vi "Configure Dialog.vi"(8 "error in (no error)":errorcluster, 11 "Configure Sparse Marker [SM] Msg.lvclass":refnum<class "Configure Sparse Marker [SM] Msg.lvclass">) -> (0 "error out":errorcluster, 2 "Ok?":bool, 3 "Configure Sparse Marker [SM] Msg.lvclass":refnum<class "Configure Sparse Marker [SM] Msg.lvclass">)   [LabVIEW 2015, in "CS++Fgen.lvlib" / "Configure Sparse Marker [SM] Msg.lvclass"]
uses:
  Configure Sparse Marker [SM] Msg.lvclass
  Configure Sparse Marker [SM] Msg.lvclass/Configure Sparse Marker [SM] Msg.ctl
panel:
  in  "Indexes Array":i64[](array[numeric])
  in  "Cancel Button":bool
  in  "OK Button":bool
  in  "Destination Terminal":string
  in  "Marker Name":string
  in  "Number Indexes":i64
  in  "Waveform Handle":i32
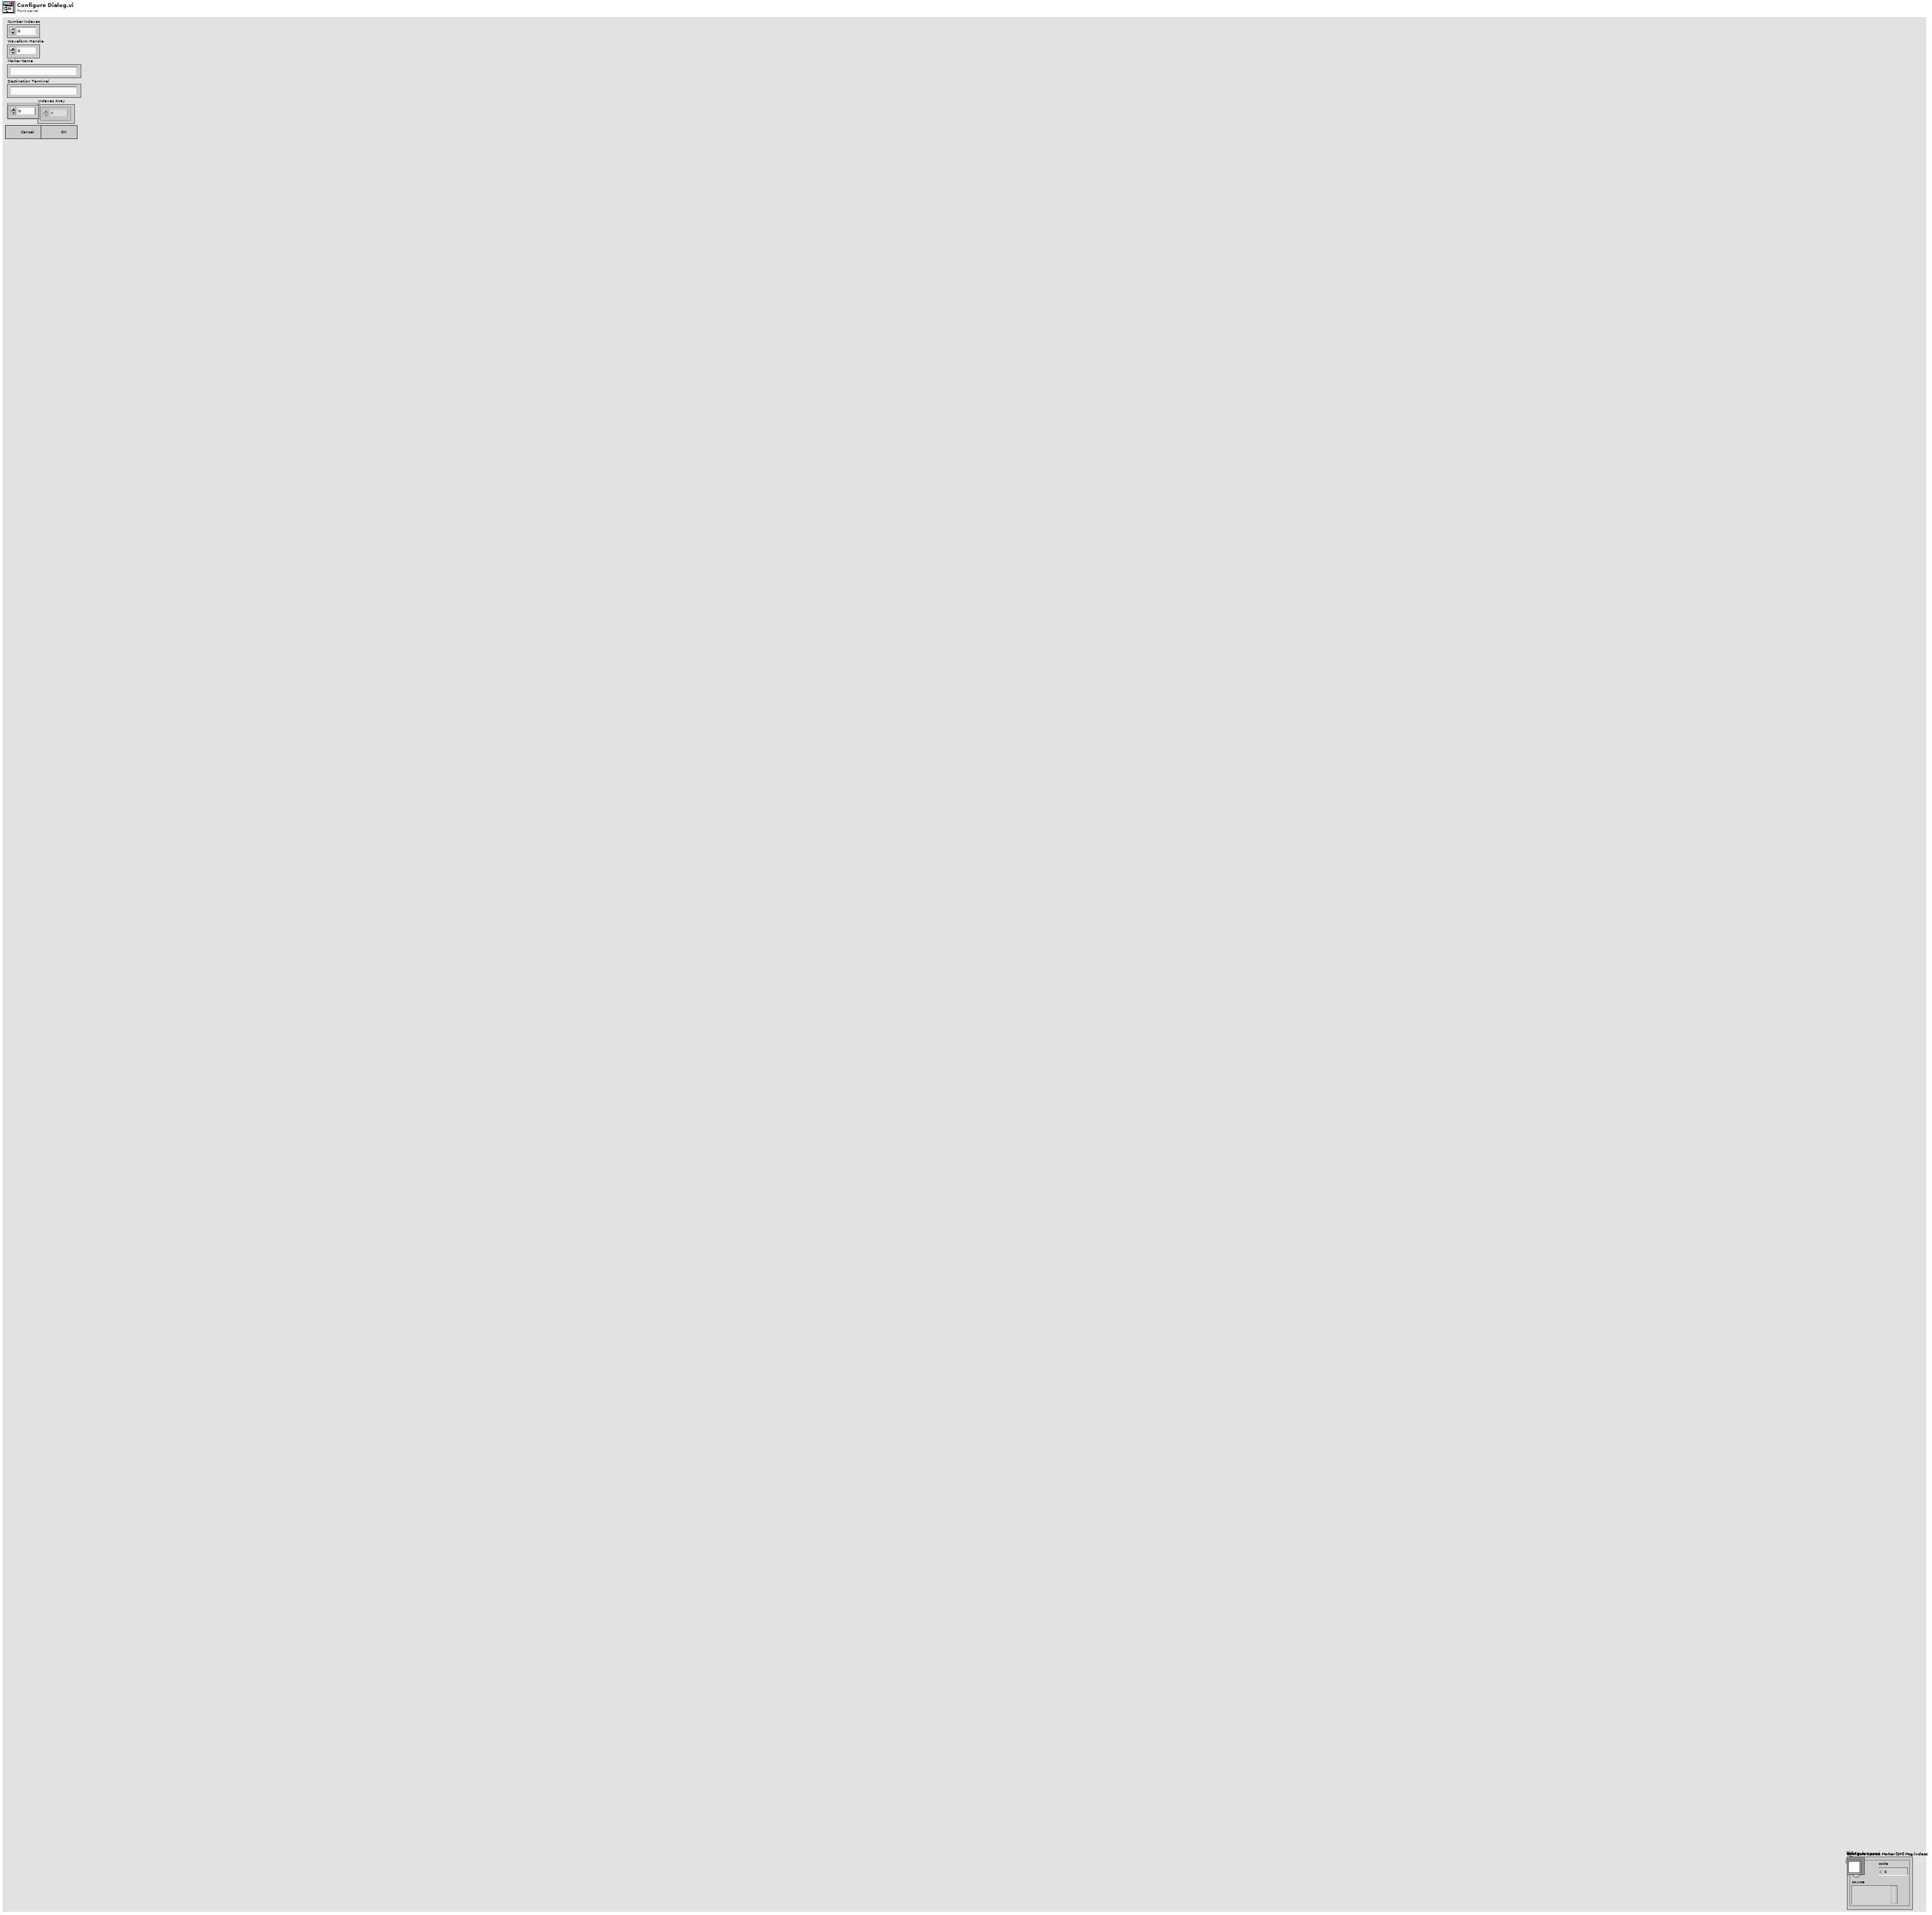
[diagram p1: front panel]
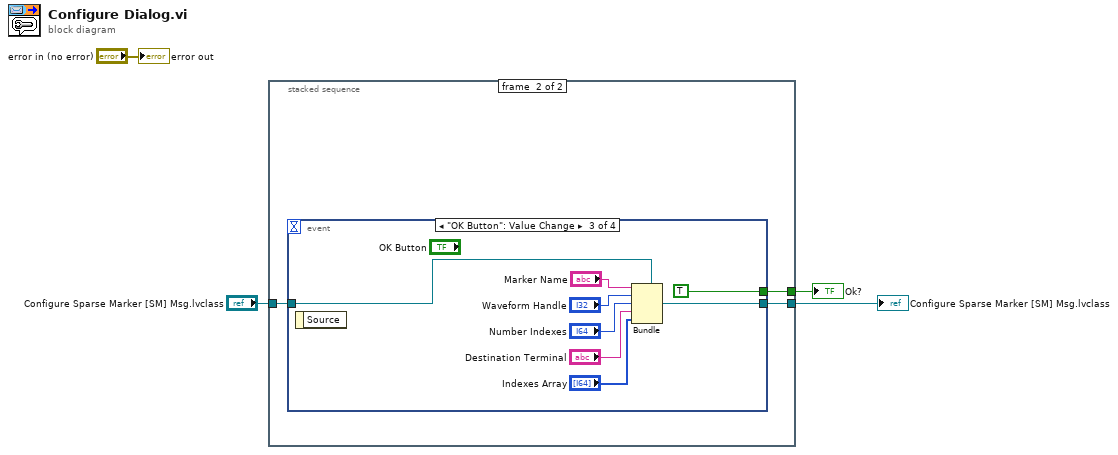
[diagram p0: block diagram]
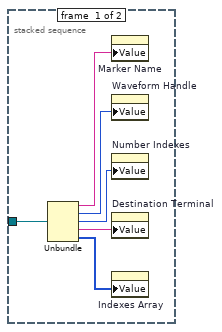
[diagram p2: hidden frame]
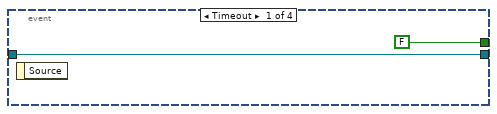
[diagram p3: hidden frame]
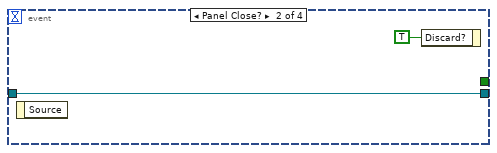
[diagram p4: hidden frame]
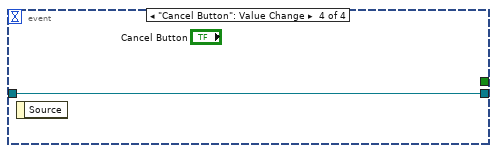
[diagram p5: hidden frame]
diagram:
  n1 = stacked-sequence {
    tunnel: [_ w13] -> w3
    tunnel: [_ w12] -> w2
    tunnel: "Configure Sparse Marker [SM] Msg.lvclass" -> [w10 w11]
    frame #0 {
      n2 = Unbundle ("Seq0Unbundler")(w10) -> (w9:string, w8:i32, w7:i64, w6:string, w5:i64[])
      n3 = property on="Marker Name" class="Str"("Value"=w9) -> ()  [unwired: 2 in, 2 out]
      n4 = property on="Waveform Handle" class="DigNum (strict)"("Value"=w8) -> ()  [unwired: 2 in, 2 out]
      n5 = property on="Number Indexes" class="DigNum (strict)"("Value"=w7) -> ()  [unwired: 2 in, 2 out]
      n6 = property on="Destination Terminal" class="Str"("Value"=w6) -> ()  [unwired: 2 in, 2 out]
      n7 = property on="Indexes Array" class="Arr (strict)"("Value"=w5) -> ()  [unwired: 2 in, 2 out]
    }
    frame #1 {
      n8 = event shown="[2] \"OK Button\": Value Change" {
        selector: _ -> [_ _ _ _]
        dyn-events: _ -> [_ _ _ _]
        timeout: _ -> [_ _ _ _]
        tunnel: [w14 w16 w23 w26] -> w12
        tunnel: w11 -> [w14 w16 w25 w26]
        tunnel: [FALSE _ TRUE _] -> w13
        event Timeout {
          n9 = event-data() -> ()  [unwired: 1 in, 1 out]
        }
        event Panel Close? {
          n10 = event-data() -> ()  [unwired: 1 in, 1 out]
          n11 = event-data ("Event Filter Node")("Discard?"=TRUE) -> ()  [unwired: 1 in, 1 out]
        }
        event "OK Button": Value Change {
          n12 = event-data() -> ()  [unwired: 1 in, 1 out]
          n13 = Bundle ("Main-Bundler")(cluster=w25, "Marker Name", "Waveform Handle", "Number Indexes", "Destination Terminal", "Indexes Array") -> (w23:refnum<class "Configure Sparse Marker [SM] Msg.lvclass">)
        }
        event "Cancel Button": Value Change {
          n14 = event-data() -> ()  [unwired: 1 in, 1 out]
        }
      }
    }
  }
  "Ok?" <- w3
  "Configure Sparse Marker [SM] Msg.lvclass" <- w2
  "error out" <- "error in (no error)"
